vi "Close Measurement.vi"(8 "error in":errorcluster, 11 "gRPCid in":u64) -> (0 "error out":errorcluster)   [LabVIEW 2021, in "Measurement Client Template.lvlib"]
doc: "Close the measurement client connection."
uses:
  Measurement Client Template.lvlib
  <vilib>/gRPC/Generated APIs/ni/measurementlink/measurement/v2/Measurement Service Client V2/Measurement Service Client V2.lvlib
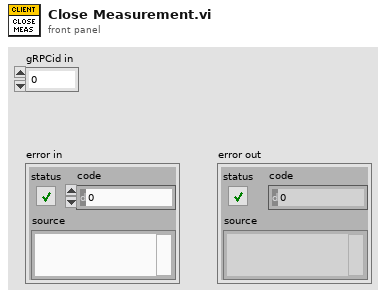
[diagram p1: front panel]
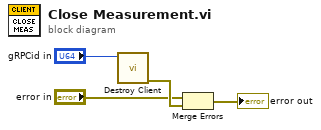
[diagram p0: block diagram]
diagram:
  n1 = call <vilib>:"Destroy Client.vi"("gRPC ID"="gRPCid in") -> ("error out"=w3:errorcluster)  [unwired: 10 in]
  n2 = Merge Errors("error in", w3) -> (→"error out":errorcluster)
